vi "Index Joint Trajectory.vi"(10 "Index":i32, 11 "Trajectory Cluster":T1) -> (3 "Indexed Joint Posit":dbl[](array[numeric]))   [LabVIEW 2016]
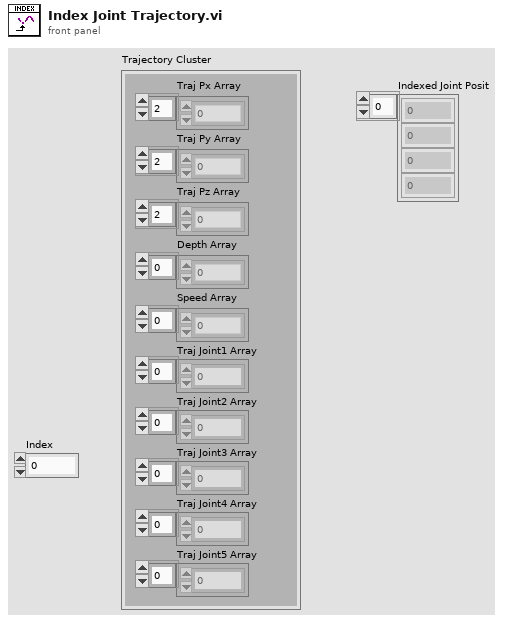
[diagram p1: front panel]
types:
  T1 = cluster{"Traj Px Array":dbl[], "Traj Py Array":dbl[], "Traj Pz Array":dbl[], "Speed Array":dbl[], "Depth Array":dbl[], "Traj Joint1 Array":dbl[], "Traj Joint2 Array":dbl[], "Traj Joint3 Array":dbl[], "Traj Joint4 Array":dbl[], "Traj Joint5 Array":dbl[]}
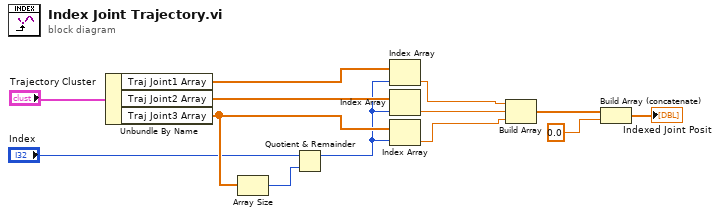
[diagram p0: block diagram]
diagram:
  n1 = Unbundle By Name("Trajectory Cluster") -> ("Traj Joint1 Array"=w9:dbl[], "Traj Joint2 Array"=w13:dbl[], "Traj Joint3 Array"=w7:dbl[])
  n2 = Array Size(array=w7) -> (size(s)=w6:i32)
  n3 = Quotient & Remainder(x="Index", y=w6) -> (x-y*floor(x/y)=w5:i32)  [unwired: 1 out]
  n4 = Index Array(array=w9, index=w5) -> (element=w12:dbl)
  n5 = Index Array(array=w13, index=w5) -> (element=w11:dbl)
  n6 = Index Array(array=w7, index=w5) -> (element=w10:dbl)
  n7 = Build Array(w12, w11, w10) -> (w1:dbl[])
  n8 = Build Array (concatenate)(w1, 0.0 ("element")) -> (→"Indexed Joint Posit":dbl[])
